vi "Read Resource Name.vi"(8 "error in (no error)":errorcluster, 11 "Power Detector in":refnum<class "Power Detector.lvclass">) -> (0 "error out":errorcluster, 2 "Resource Name":refnum<k15>, 3 "Power Detector out":refnum<class "Power Detector.lvclass">)   [LabVIEW 2023, in "NI CAL-5501 Power Detector.lvlib" / "Power Detector.lvclass"]
uses:
  Power Detector.lvclass
  Power Detector.lvclass/Power Detector.ctl
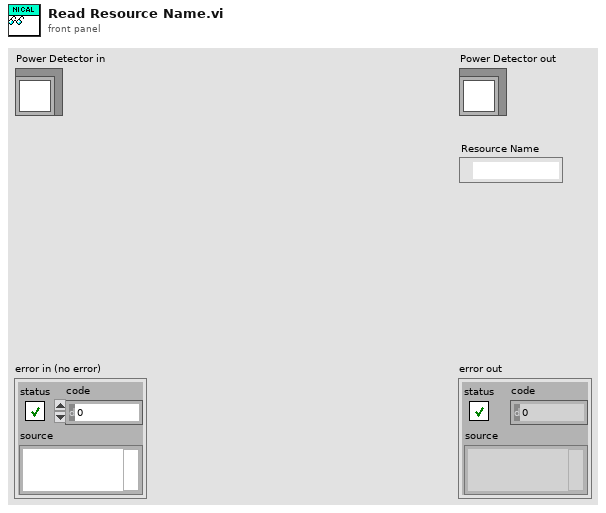
[diagram p1: front panel]
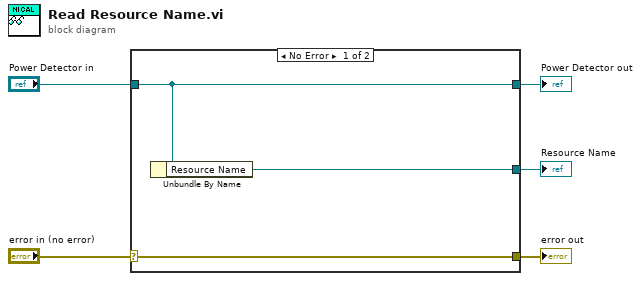
[diagram p0: block diagram]
diagram:
  n1 = case shown="No Error" "error in (no error)" {
    selector: "error in (no error)" -> [w8 w9]
    tunnel: [w8 w9] -> w4
    tunnel: [w7 w10] -> w2
    tunnel: "Power Detector in" -> [w7 w10]
    tunnel: [w6 _] -> w1
    frame No Error {
      n2 = Unbundle By Name(w7) -> ("Resource Name"=w6:refnum<k15>)
    }
    frame Error {
    }
  }
  "error out" <- w4
  "Power Detector out" <- w2
  "Resource Name" <- w1
